vi "Delta T.vi"(8 "Background":dbl[][](array[numeric]), 9 "FrameData":dbl[][][](array[numeric])) -> (0 "FrameData even":dbl[][][](array[numeric]), 1 "FrameData odd":dbl[][][](array[numeric]), 2 "Delta T":dbl[][](array[numeric]), 3 "Delta T over T":dbl[][](array[numeric]))   [LabVIEW 2020]
uses:
  Random subVIs/Control 1.ctl
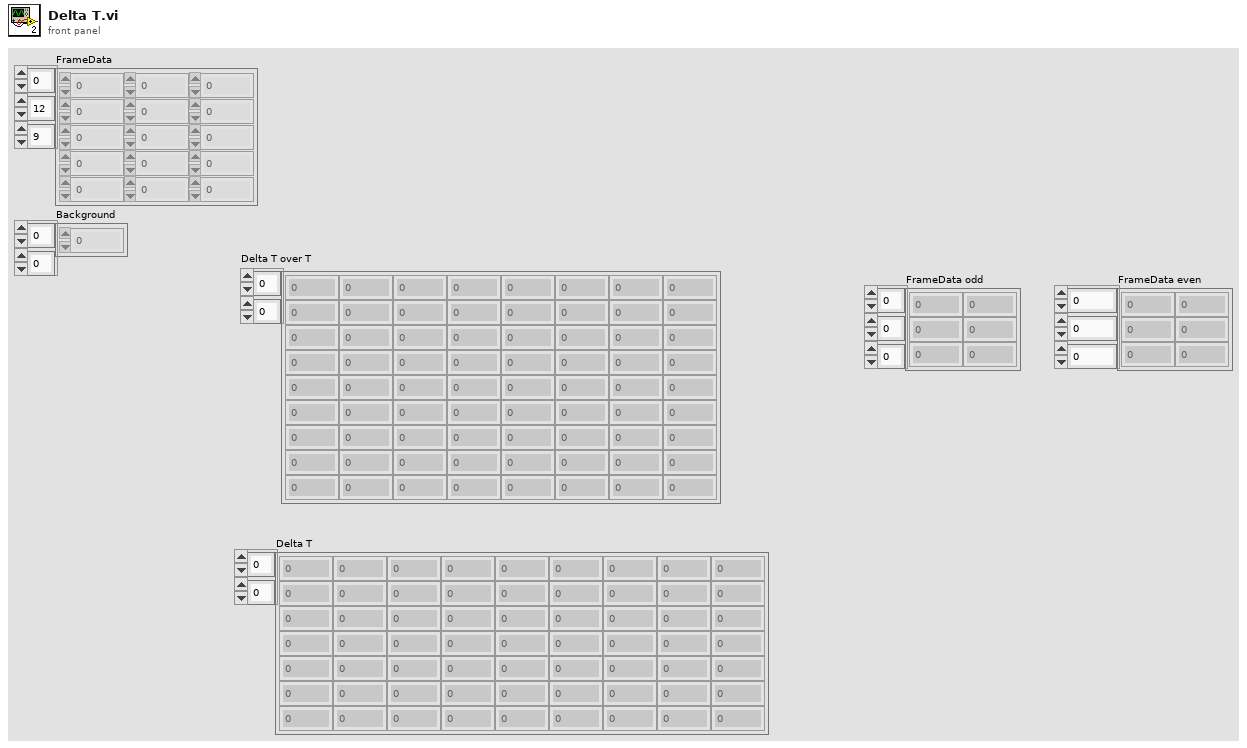
[diagram p1: front panel]
types:
  T1 = typedef "Control 1.ctl" = i32
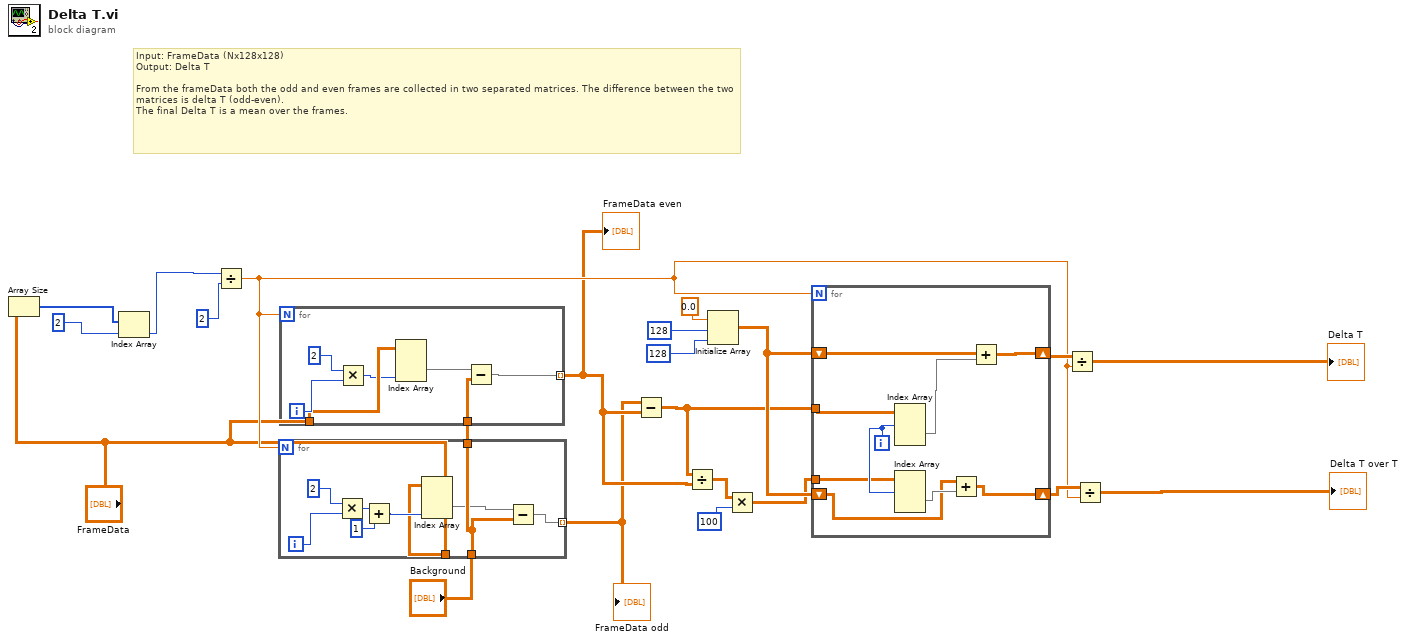
[diagram p0: block diagram]
diagram:
  # "Input: FrameData (Nx128x128)\nOutput: Delta T\n\nFrom the frameData both the odd and even frames are collected in two separated matrices. The difference between the two matrices is delta T (odd-even). \nThe final Delta T is a mean over the frames."
  n1 = Array Size(array="FrameData") -> (size(s)=w16:i32[])
  n2 = Index Array(array=w16, index=2) -> (element=w15:i32)
  n3 = Divide(x=w15, y=T1 2) -> (x/y=w12:dbl)
  n4 = for {
    N: w12 -> [_]
    tunnel: "FrameData" -> [w26]
    tunnel: "Background" -> [w24]
    tunnel: [w25] -> w2 mode=indexing
    tunnel: [w24] -> w9
    i -> [w31]
    n5 = Multiply(x=2, y=w31) -> (x*y=w29:i32)
    n6 = Add(x=w29, y=1) -> (x+y=w27:i32)
    n7 = Index Array(array=w26, index (dim 2)=w27) -> (element=w23:dbl[][])  [unwired: 2 in]
    n8 = Subtract(x=w23, y=w24) -> (x-y=w25:dbl[][])
  }
  "FrameData odd" <- w2
  n9 = for {
    N: w12 -> [_]
    tunnel: [w33] -> w3 mode=indexing
    tunnel: "FrameData" -> [w36]
    tunnel: w9 -> [w34]
    i -> [w38]
    n10 = Multiply(x=2, y=w38) -> (x*y=w35:i32)
    n11 = Index Array(array=w36, index (dim 2)=w35) -> (element=w32:dbl[][])  [unwired: 2 in]
    n12 = Subtract(x=w32, y=w34) -> (x-y=w33:dbl[][])
  }
  "FrameData even" <- w3
  n13 = Subtract(x=w2, y=w3) -> (x-y=w10:dbl[][][])
  n14 = Divide(x=w10, y=w3) -> (x/y=w8:dbl[][][])
  n15 = Initialize Array(0.0 ("element"), 128 ("dimension size"), 128 ("dimension size")) -> (w14:dbl[][])
  n16 = Multiply(x=w8, y=100) -> (x*y=w7:dbl[][][])
  n17 = for {
    N: w12 -> [_]
    tunnel: w10 -> [w47]
    shift-right: [w45] -> w18
    shift-left: w14 -> [w40]
    shift-right: [w42] -> w13
    shift-left: w14 -> [w39]
    tunnel: w7 -> [w41]
    i -> [w44]
    n18 = Index Array(array=w47, index (dim 0)=w44) -> (element=w46:dbl[][])  [unwired: 2 in]
    n19 = Index Array(array=w41, index (dim 0)=w44) -> (element=w43:dbl[][])  [unwired: 2 in]
    n20 = Add(x=w39, y=w43) -> (x+y=w42:dbl[][])
    n21 = Add(x=w40, y=w46) -> (x+y=w45:dbl[][])
  }
  n22 = Divide(x=w18, y=w12) -> (x/y=→"Delta T":dbl[][])
  n23 = Divide(x=w13, y=w12) -> (x/y=→"Delta T over T":dbl[][])
